vi "SR400 SetGateParams.vi"(6 "error in (no error)":errorcluster, 7 "BGatePar":T1={"Mode"=0, "Durée"=0.9992, "Délais"=0.9992, "Incrément"=0.9992} caption="Paramètres de la porte d'acquisition «B»" {"Incrément" min=0.0 max=0.9992 step=1e-09 format="%#_4g"; "Délais" min=0.0 max=0.9992 step=1e-09 format="%#_4g"; "Durée" min=5e-09 max=0.9992 step=1e-09 format="%#_4g"; "Mode" items=["CW", "Fixed", "Scan"]}, 8 "AGatePar":T1={"Mode"=0, "Durée"=0.9992, "Délais"=0.9992, "Incrément"=0.9992} caption="Paramètres de la porte d'acquisition «A»" {"Incrément" min=0.0 max=0.9992 step=1e-09 format="%#_4g"; "Délais" min=0.0 max=0.9992 step=1e-09 format="%#_4g"; "Durée" min=5e-09 max=0.9992 step=1e-09 format="%#_4g"; "Mode" items=["CW", "Fixed", "Scan"]}, 9 "VISA Port In":refnum<visa-resource-name>="GPIB0::23::INSTR") -> (0 "error out":errorcluster, 3 "VISA Port Out":refnum<visa-resource-name>="GPIB0::23::INSTR")   [LabVIEW 2012]
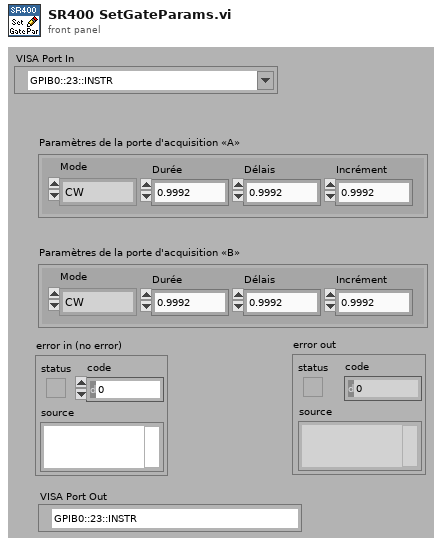
[diagram p1: front panel]
types:
  T1 = cluster{"Mode":u16, "Durée":dbl, "Délais":dbl, "Incrément":dbl}
  T2 = enum16{"Lit le Statut", "Configure", "Oper. incomp."}
  T3 = cluster{"Mode":u16, "Durée":dbl, "Délais":dbl, "Incrément":dbl}[]
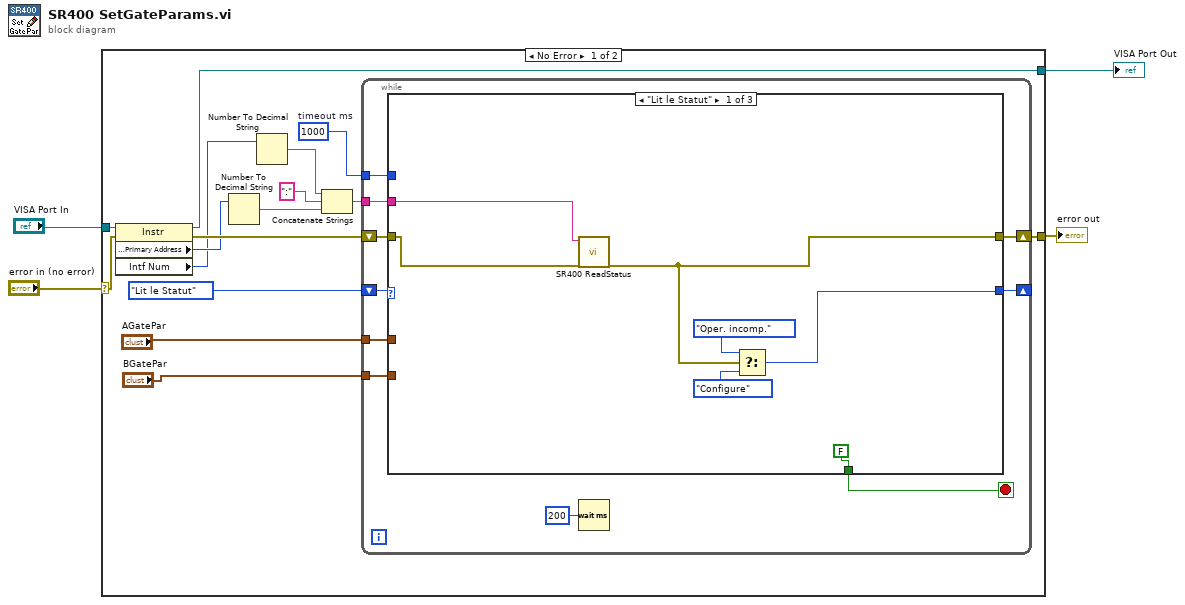
[diagram p0: block diagram]
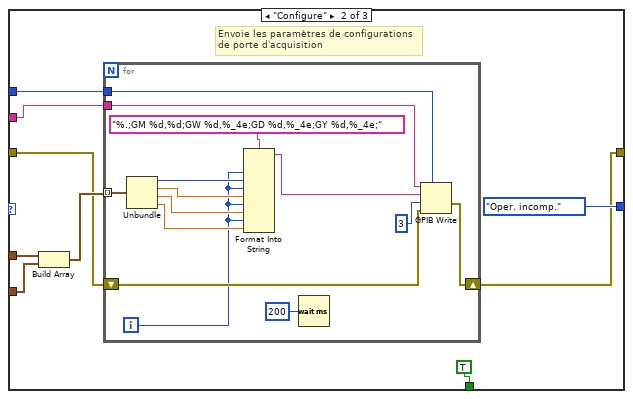
[diagram p2: hidden frame]
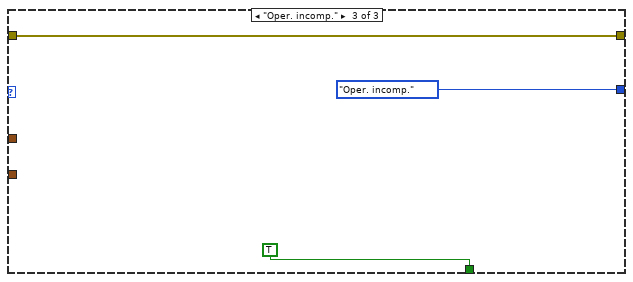
[diagram p3: hidden frame]
diagram:
  n1 = case shown="No Error" "error in (no error)" {
    selector: "error in (no error)" -> [w19 w64]
    tunnel: [w13 w64] -> w3
    tunnel: "VISA Port In" -> [w18 w63]
    tunnel: [w5 w63] -> w1
    frame No Error {
      w14 = 1000  # timeout ms
      n2 = property class="Instr"(reference=w18, error in=w19) -> (reference out=w5:refnum<visa-resource-name>, error out=w17:errorcluster, "GPIB Settings:Primary Address"=w15:u16, "Intf Num"=w10:u16)
      n3 = Number To Decimal String(number=w15) -> (decimal integer string=w8:string)  [unwired: 1 in]
      n4 = Number To Decimal String(number=w10) -> (decimal integer string=w9:string)  [unwired: 1 in]
      n5 = Concatenate Strings(w9, ":" ("string"), w8) -> (w6:string)
      n6 = while {
        shift-right: [w23] -> _
        shift-left: T2."Lit le Statut" -> [w29]
        tunnel: w6 -> [w27]
        shift-right: [w26] -> w13
        shift-left: w17 -> [w28]
        tunnel: w14 -> [w25]
        tunnel: "AGatePar" -> [w21]
        tunnel: "BGatePar" -> [w20]
        stop <- w24 stop-if-true
        n7 = case shown="\"Lit le Statut\"" w29 {
          tunnel: w28 -> [w35 w41 w62]
          tunnel: w27 -> [w34 w39 _]
          tunnel: [w30 w37 w62] -> w26
          tunnel: w25 -> [_ w38 _]
          tunnel: [FALSE ("Configuration\neffectuée") TRUE ("Configuration\neffectuée") TRUE ("Configuration\neffectuée")] -> w24
          tunnel: [w31 T2."Oper. incomp." T2."Oper. incomp."] -> w23
          tunnel: w21 -> [_ w44 _]
          tunnel: w20 -> [_ w43 _]
          frame "Lit le Statut" {
            n8 = call <userlib>:"SR400 ReadStatus.vi"("error in"=w35, "Address string"=w34) -> ("Error Out"=w30:errorcluster)  [unwired: 6 in, 1 out]
            n9 = Select(t=T2."Oper. incomp.", s=w30, f=T2."Configure") -> (s? t:f=w31:T2)
          }
          frame "Configure" {
            # "Envoie les paramètres de configurations de porte d'acquisition"
            n10 = Build Array(w44, w43) -> (w42:T3)
            n11 = for {
              tunnel: w42 -> [w58] mode=indexing
              shift-right: [w56] -> w37
              shift-left: w41 -> [w57]
              tunnel: w39 -> [w55]
              tunnel: w38 -> [w54]
              i -> [w47]
              n12 = Unbundle(w58) -> ("Mode"=w51:u16, "Durée"=w50:dbl, "Délais"=w48:dbl, "Incrément"=w49:dbl)
              n13 = Format Into String(format string="%.;GM %d,%d;GW %d,%_4e;GD %d,%_4e;GY %d,%_4e;", w47, w51, w47, w50, w47, w48, w47, w49) -> (resulting string=w46:string)  [unwired: 2 in, 1 out]
              n14 = Wait (ms)(milliseconds to wait=u32 200) -> ()  [unwired: 1 out]
              n15 = GPIB Write(0:w55, 1:w46, 2:i16 3 ("mode (0)"), 3:w57, 4:w54) -> (6:w56:errorcluster)  [unwired: 1 out]
            }
          }
          frame "Oper. incomp." {
          }
        }
        n16 = Wait (ms)(milliseconds to wait=u32 200) -> ()  [unwired: 1 out]
      }
    }
    frame Error {
    }
  }
  "error out" <- w3
  "VISA Port Out" <- w1
